vi "Modbus Visa.vi"(1 "VISA resource name":refnum<visa-resource-name>, 2 "Cmd":string, 3 "TimeOut":bool=TRUE, 4 "Time(0.1)":u32=10, 5 "error in (no error)":errorcluster, 8 "VisaAction":enum16{"Open", "Send", "Recieve", "Close"}(ring)) -> (16 "read string":string, 19 "error out":errorcluster)   [LabVIEW 2019]
uses:
  <vilib>/Instr/_visa.llb/VISA Configure Serial Port (Instr).vi
  LLB/Commonly VI.lvlib
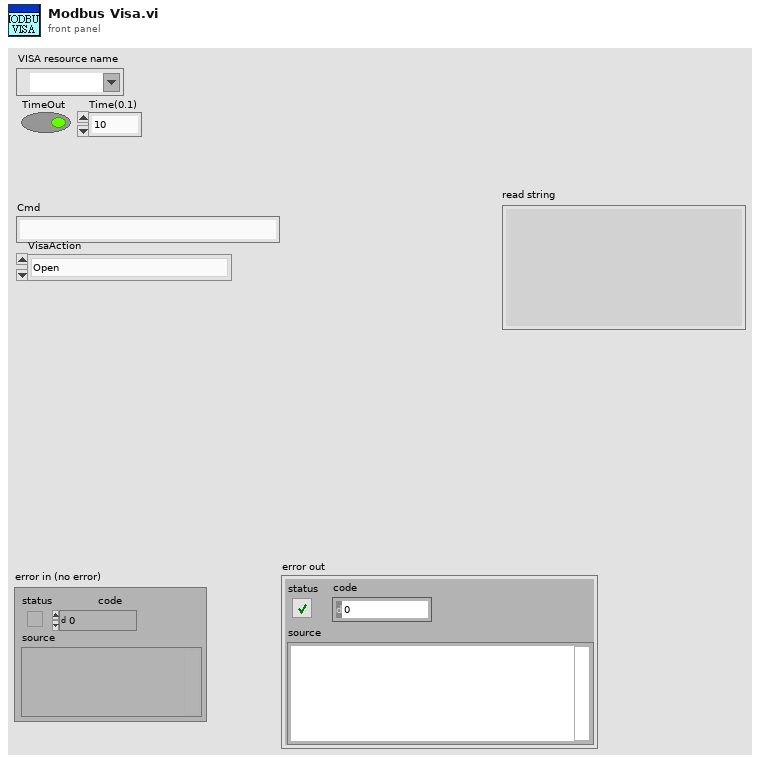
[diagram p1: front panel]
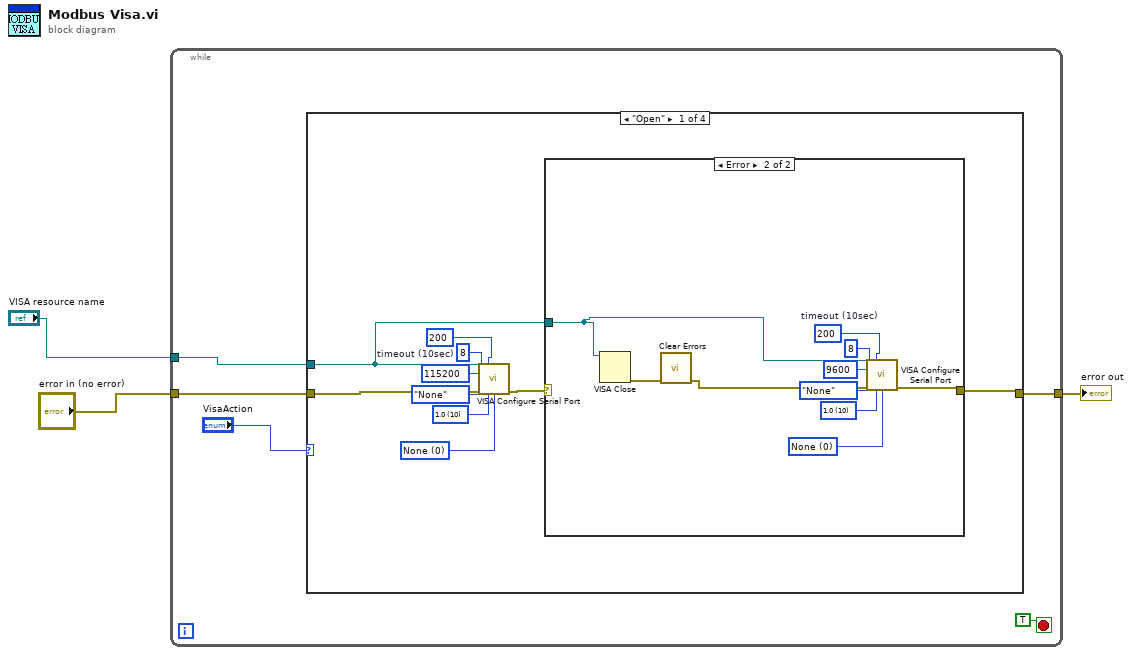
[diagram p0: block diagram]
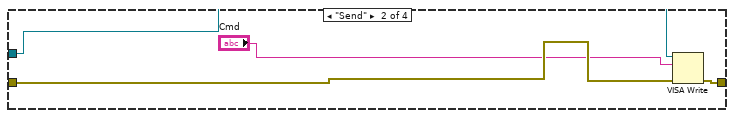
[diagram p3: hidden frame]
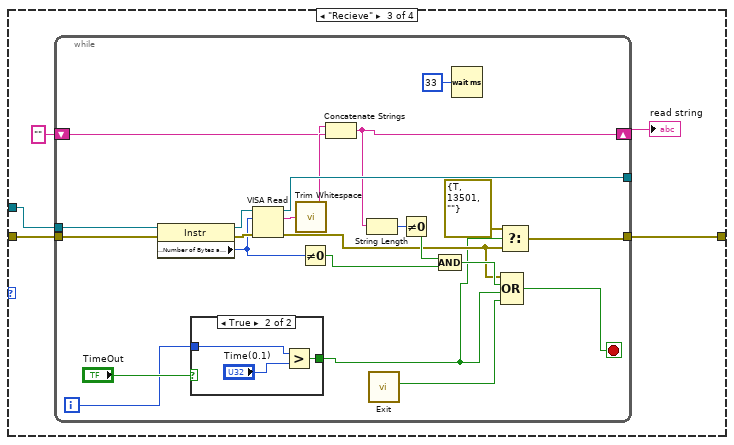
[diagram p4: hidden frame]
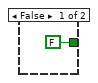
[diagram p5: hidden frame]
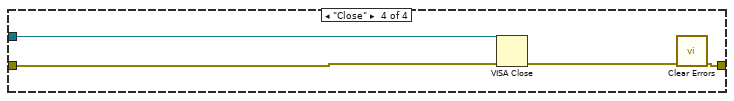
[diagram p6: hidden frame]
diagram:
  n1 = while {
    tunnel: "error in (no error)" -> [w6]
    tunnel: [w7] -> w3
    tunnel: "VISA resource name" -> [w4]
    stop <- TRUE stop-if-true
    n2 = case shown="\"Open\"" "VisaAction" {
      tunnel: [w10 w33 w37 w67] -> w7
      tunnel: w6 -> [w18 w32 w38 w68]
      tunnel: w4 -> [w9 w31 w34 w66]
      frame "Open" {
        w13 = u16 0 items=["None", "XON/XOFF", "RTS/CTS", "XON/XOFF & RTS/CTS", "DTR/DSR", "XON/XOFF & DTR/DSR"] ("flow control (0:none)")
        w14 = u16 10 items=["1.0"=10, "1.5"=15, "2.0"=20] ("stop bits (10: 1 bit)")
        w17 = u32 200  # timeout (10sec)
        n3 = call-poly "VISA Configure Serial Port"("VISA resource name"=w9, "timeout (10sec)"=w17, "baud rate (9600)"=u32 115200, "data bits (8)"=u16 8, "parity (0:none)"=enum16{"None", "Odd", "Even", "Mark", "Space"}."None", "error in (no error)"=w18, "stop bits (10: 1 bit)"=w14, "flow control (0:none)"=w13) -> ("error out"=w11:errorcluster)  [unwired: 1 in, 6 out]
        n4 = case shown="Error" w11 {
          selector: w11 -> [w19 _]
          tunnel: [w19 w20] -> w10
          tunnel: w9 -> [_ w21]
          frame No Error {
          }
          frame Error {
            w28 = u16 0 items=["None", "XON/XOFF", "RTS/CTS", "XON/XOFF & RTS/CTS", "DTR/DSR", "XON/XOFF & DTR/DSR"] ("flow control (0:none)")
            w27 = u16 10 items=["1.0"=10, "1.5"=15, "2.0"=20] ("stop bits (10: 1 bit)")
            w24 = u32 200  # timeout (10sec)
            n5 = VISA Close(VISA resource name=w21) -> (error out=w23:errorcluster)  [unwired: 1 in]
            n6 = call <vilib>:"Clear Errors.vi"("error in (no error)"=w23) -> ("error out"=w22:errorcluster)  [unwired: 5 in, 1 out]
            n7 = call-poly "VISA Configure Serial Port"("VISA resource name"=w21, "timeout (10sec)"=w24, "baud rate (9600)"=u32 9600, "data bits (8)"=u16 8, "parity (0:none)"=enum16{"None", "Odd", "Even", "Mark", "Space"}."None", "error in (no error)"=w22, "stop bits (10: 1 bit)"=w27, "flow control (0:none)"=w28) -> ("error out"=w20:errorcluster)  [unwired: 1 in, 6 out]
          }
        }
      }
      frame "Send" {
        n8 = VISA Write(VISA resource name=w31, write buffer="Cmd", error in (no error)=w32) -> (error out=w33:errorcluster)  [unwired: 2 out]
      }
      frame "Recieve" {
        n9 = while {
          tunnel: w38 -> [w59]
          tunnel: [w58] -> _
          tunnel: [w53] -> w37
          shift-right: [w50] -> w36
          shift-left: "" ("trimmed string") -> [w56]
          tunnel: w34 -> [w39]
          i -> [w42]
          stop <- w54 stop-if-true
          n10 = property class="Instr"(reference=w39, error in=w59) -> (reference out=w60:refnum<visa-resource-name>, error out=w61:errorcluster, "Serial Settings:Number of Bytes at Serial Port"=w43:u32)
          n11 = case shown="True" "TimeOut" {
            tunnel: w42 -> [_ w65]
            tunnel: [FALSE w63] -> w41
            frame False {
            }
            frame True {
              n12 = Greater?(x=w65, y="Time(0.1)") -> (0:w63:bool)
            }
          }
          n13 = VISA Read(VISA resource name=w60, byte count=w43, error in (no error)=w61) -> (VISA resource name out=w58:refnum<visa-resource-name>, read buffer=w45:string, error out=w46:errorcluster)  [unwired: 1 out]
          n14 = call <vilib>:"Trim Whitespace.vi"("string"=w45) -> ("trimmed string"=w57:string)  [unwired: 1 in]
          n15 = Not Equal To 0?(x=w43) -> (x != 0?=w51:bool)
          n16 = Concatenate Strings(w56, w57) -> (w50:string)
          n17 = String Length(string=w50) -> (length=w49:i32)
          n18 = call "Exit.vi"() -> ("ExitOut"=w40:bool)  [unwired: 11 in]
          n19 = Not Equal To 0?(x=w49) -> (x != 0?=w48:bool)
          n20 = Compound Arithmetic op=AND(w48, w51) -> (w47:bool)
          n21 = Wait (ms)(milliseconds to wait=u32 33) -> ()  [unwired: 1 out]
          n22 = Select(t=errorcluster {"status"=TRUE, "code"=13501, "source"=""}, s=w41, f=w46) -> (s? t:f=w53:errorcluster)
          n23 = Compound Arithmetic op=OR(w46, w47, w41, w40) -> (w54:bool)
        }
        "read string" <- w36
      }
      frame "Close" {
        n24 = VISA Close(VISA resource name=w66, error in (no error)=w68) -> (error out=w69:errorcluster)
        n25 = call <vilib>:"Clear Errors.vi"("error in (no error)"=w69) -> ("error out"=w67:errorcluster)  [unwired: 5 in, 1 out]
      }
    }
  }
  "error out" <- w3
